vi "agilent_34970A_resistances(real)-error.vi"(4 "error in (no error)":errorcluster, 5 "Channels":string, 6 "Readings":u16=1, 7 "Agilent Port In":refnum<visa-resource-name>="COM35") -> (0 "error out":errorcluster, 1 "Res StnDev":dbl[](array[numeric]), 2 "Resistances":dbl[](array[numeric]), 3 "Agilent Port Out":refnum<visa-resource-name>="COM35")   [LabVIEW 2010]
uses:
  <vilib>/Analysis/NI_AALBase.lvlib
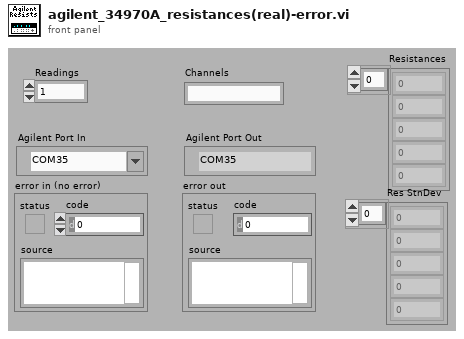
[diagram p1: front panel]
types:
  T1 = enum16{"Enable Register", "Event Register", "Operation Complete Bit"}
  T2 = enum16{"Manual", "Minimum", "Maximum", "Infinity"}
  T3 = enum16{"Bus", "Immediate", "External", "Alarm 1", "Alarm 2", "Alarm 3", "Alarm 4", "Timer"}
  T4 = cluster{"Include Alarm Data? (F:No)":bool, "Include Channel #? (F:No)":bool, "Include Time? (F:No)":bool, "Include Units? (F:No)":bool}
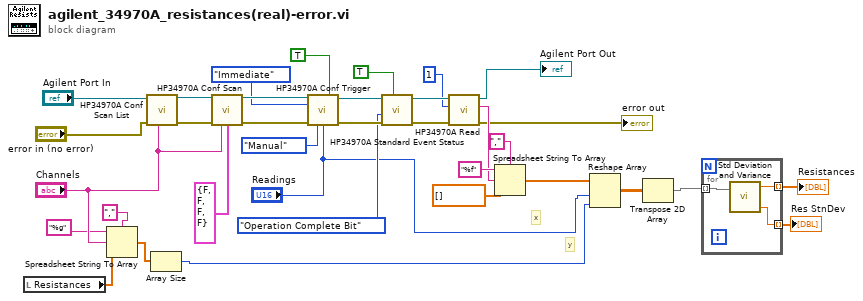
[diagram p0: block diagram]
diagram:
  # "y"
  # "x"
  n1 = local read "Resistances"() -> (w6:dbl[])
  n2 = Spreadsheet String To Array(delimiter (Tab)=",", format string="%g", spreadsheet string="Channels", array type (2D Dbl)=w6) -> (array=w7:dbl[])
  n3 = call "HP34970A Conf Scan List.vi"("Scan List (empty)"="Channels", "error in (no error)"="error in (no error)", "VISA resource name"="Agilent Port In") -> ("error out"=w32:errorcluster, "VISA resource name out"=w33:refnum<visa-resource-name>)  [unwired: 6 in, 1 out]
  n4 = Array Size(array=w7) -> (size(s)=w5:i32)
  n5 = call "HP34970A Conf Scan.vi"("VISA resource name"=w33, "error in (no error)"=w32, "Channel List (empty)"="Channels", "Scan Fields"=T4 {"Include Alarm Data? (F:No)"=FALSE, "Include Channel #? (F:No)"=FALSE, "Include Time? (F:No)"=FALSE, "Include Units? (F:No)"=FALSE}) -> ("VISA resource name out"=w30:refnum<visa-resource-name>, "error out"=w29:errorcluster)  [unwired: 9 in, 1 out]
  n6 = call "HP34970A Conf Trigger.vi"("VISA resource name"=w30, "Wait for Trigger? (F:No)"=TRUE, "Source (1:Immediate)"=T3."Immediate", "error in (no error)"=w29, "Max Trigger Count (3:Inf)"=T2."Manual", "# Triggers (1)"="Readings") -> ("VISA resource name out"=w25:refnum<visa-resource-name>, "error out"=w24:errorcluster)  [unwired: 7 in, 1 out]
  n7 = call "HP34970A Standard Event Status.vi"("Set/Check? (F:Set)"=TRUE, "error in (no error)"=w24, "Check Parameter (0:Enable Reg)"=T1."Operation Complete Bit", "VISA resource name"=w25) -> ("error out"=w35:errorcluster, "VISA resource name out"=w34:refnum<visa-resource-name>)  [unwired: 5 in, 1 out]
  n8 = call "HP34970A Read.vi"("error in (no error)"=w35, "# Channels (1)"=1, "VISA resource name"=w34) -> ("error out"=→"error out":errorcluster, "Readings"=w16:string, "VISA resource name out"=→"Agilent Port Out":refnum<visa-resource-name>)  [unwired: 5 in, 1 out]
  n9 = Spreadsheet String To Array(delimiter (Tab)=",", format string="%f", spreadsheet string=w16, array type (2D Dbl)=dbl[] []) -> (array=w12:dbl[])
  n10 = Reshape Array(w12, "Readings", w5) -> (w13:dbl[][])
  n11 = Transpose 2D Array(2D array=w13) -> (transposed array=w10:dbl[][])
  n12 = for {
    tunnel: w10 -> [w38] mode=indexing
    tunnel: [w37] -> w9 mode=indexing
    tunnel: [w36] -> w8 mode=indexing
    n13 = call <vilib>:"Std Deviation and Variance.vi"("X"=w38) -> ("mean"=w37:dbl, "variance"=w36:dbl)  [unwired: 1 in, 1 out]
  }
  "Resistances" <- w9
  "Res StnDev" <- w8
